vi "Frequency_Counter_BK_SoftFP.vi"(0 "reference in":refnum<class "Frequency_Counter_BK.lvclass">, 2 "Floating":bool, 5 "error in (no error)":errorcluster) -> (14 "reference out":refnum<class "Frequency_Counter_BK.lvclass">, 19 "error out":errorcluster)   [LabVIEW 2022 SP3, in "Frequency_Counter_BK.lvlib" / "Frequency_Counter_BK.lvclass"]
uses:
  Frequency_Counter_BK.lvclass
  Components/ViPER.lvlibp/ViPER.lvclass
  C:/Projects/Medulla/ViPER/Examples/Flux_Capacitor_Tester/Components/ViPER.lvlibp/ViPER.lvclass
panel:
  in  "Connect":bool
  out "Freq MHz":dbl format="%.4f"
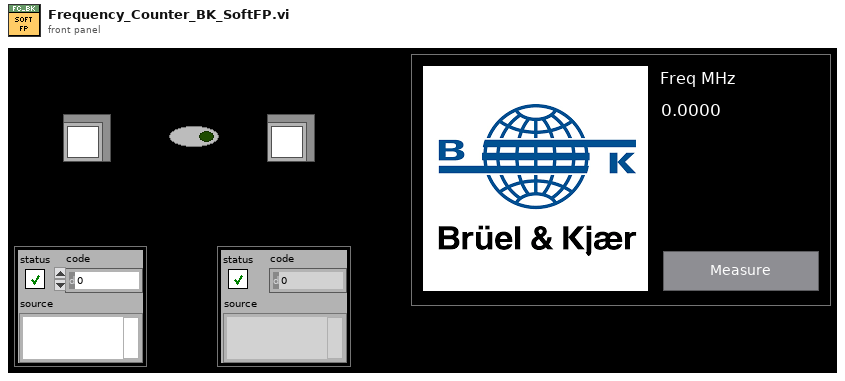
[diagram p1: front panel]
types:
  T1 = enum32{"Invalid", "Standard", "Closed", "Hidden", "Minimized", "Maximized"}
  T2 = typedef "Frequency_Counter_BK.lvlib/Frequency_Counter_BK.lvclass/ObjectAttributes.ctl" = cluster{"Config":T3, "Freq":dbl}
  T3 = typedef "Frequency_Counter_BK.lvlib/Frequency_Counter_BK.lvclass/Config.ctl" = cluster{"ComPort":refnum<visa-resource-name>, "Function":i8, "Gate_Time":i8}
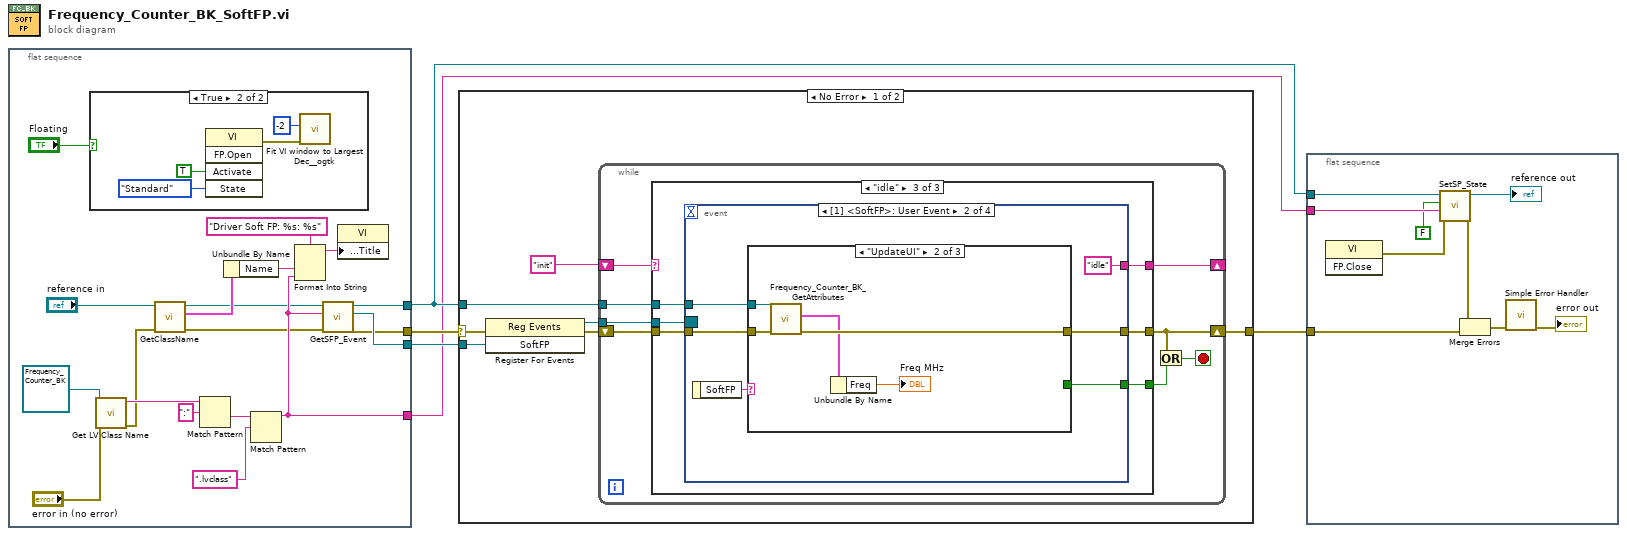
[diagram p0: block diagram]
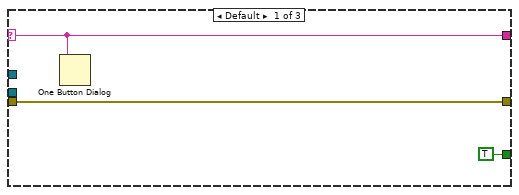
[diagram p3: hidden frame]
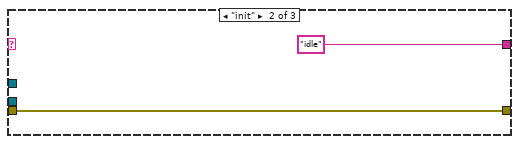
[diagram p4: hidden frame]
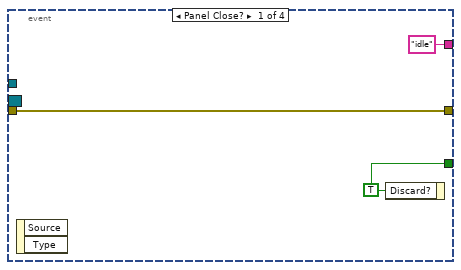
[diagram p5: hidden frame]
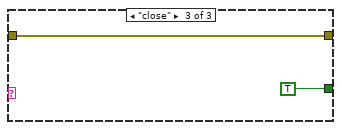
[diagram p7: hidden frame]
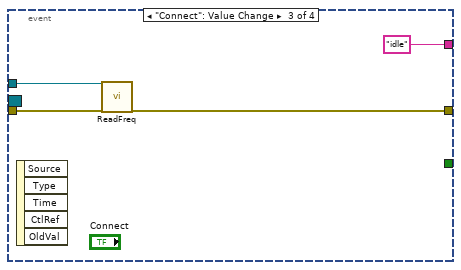
[diagram p8: hidden frame]
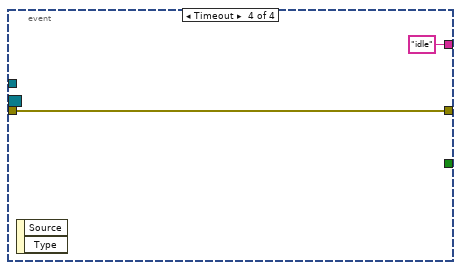
[diagram p9: hidden frame]
diagram:
  n1 = flat-sequence {
    tunnel: [w21] -> w5
    tunnel: [w20] -> w2
    tunnel: [w24] -> w3
    tunnel: [w12] -> w1
    frame #0 {
      n2 = case shown="True" "Floating" {
        frame False {
        }
        frame True {
          n3 = invoke class="VI" method="FP.Open"("Activate"=TRUE ("Activate?"), "State"=T1."Standard") -> (error out=w25:errorcluster)  [unwired: 3 in, 4 out]
          n4 = call <userlib>:"Fit VI window to Largest Dec__ogtk.vi"("error in (no error)"=w25, "border spacing (2 px)"=-2) -> ()  [unwired: 4 in, 2 out]
        }
      }
      n5 = call <vilib>:"Get LV Class Name.vi"("error in (no error)"="error in (no error)", "object"=refnum<class "Frequency_Counter_BK.lvclass"> refnum ("reference")) -> ("error out"=w11:errorcluster, "class name"=w17:string)  [unwired: 8 in]
      n6 = call "GetClassName.vi"("error in (no error)"=w11, "reference in"="reference in") -> ("error out"=w10:errorcluster, "Details"=w9:cluster{"Name":string, "Class":string}, "reference out"=w7:refnum<class "Frequency_Counter_BK.lvclass">)  [unwired: 7 in]
      n7 = Match Pattern(string=w17, regular expression=":") -> (after substring=w15:string)  [unwired: 1 in, 3 out]
      n8 = Unbundle By Name(w9) -> ("Name"=w19:string)
      n9 = Match Pattern(string=w15, regular expression=".lvclass") -> (before substring=w12:string)  [unwired: 1 in, 3 out]
      n10 = Format Into String(format string="Driver Soft FP: %s: %s", w19, w12) -> (resulting string=w23:string)  [unwired: 2 in, 1 out]
      n11 = call-dynamic "GetSFP_Event.vi"("error in (no error)"=w10, "Ancestor"=w12, "reference in"=w7) -> ("error out"=w21:errorcluster, "SoftFP"=w24:refnum<user-event>, "reference out"=w20:refnum<class "Frequency_Counter_BK.lvclass">)  [unwired: 6 in]
      n12 = property class="VI"("Front Panel.Title"=w23) -> ()  [unwired: 2 in, 2 out]
    }
  }
  n13 = case shown="No Error" w5 {
    selector: w5 -> [w33 w78]
    tunnel: [w29 w78] -> w4
    tunnel: w2 -> [w30 _]
    tunnel: w3 -> [w35 _]
    frame No Error {
      n14 = register-events(error in=w33, w35) -> (reference out=w34:refnum<event-registration>, error out=w32:errorcluster)  [unwired: 1 in]
      n15 = while {
        shift-right: [w40] -> w29
        shift-left: w32 -> [w43]
        tunnel: w34 -> [w42]
        tunnel: w30 -> [w41]
        shift-right: [w36] -> _
        shift-left: "init" -> [w37]
        stop <- w39 stop-if-true
        n16 = case shown="\"idle\"" w37 {
          selector: w37 -> [w44 _ _]
          tunnel: w43 -> [w45 w47 w54]
          tunnel: w42 -> [_ _ w53]
          tunnel: w41 -> [_ _ w52]
          tunnel: [w45 w47 w51] -> w40
          tunnel: [TRUE ("Discard?") _ w50] -> w38
          tunnel: [w44 "idle" w49] -> w36
          frame Default {
            n17 = One Button Dialog(message=w44) -> ()  [unwired: 1 in, 1 out]
          }
          frame "init" {
          }
          frame "idle" {
            n18 = event shown="[1] <SoftFP>: User Event" {
              selector: w53 -> [_ _ _ _]
              dyn-events: _ -> [_ _ _ _]
              timeout: _ -> [_ _ _ _]
              tunnel: w54 -> [w57 w63 w75 w77]
              tunnel: [w57 w61 w74 w77] -> w51
              tunnel: [w56 w60 _ _] -> w50
              tunnel: w52 -> [_ w58 w73 _]
              tunnel: ["idle" "idle" "idle" "idle"] -> w49
              event Panel Close? {
                w56 = TRUE ("Discard?")
                n19 = event-data() -> ()  [unwired: 1 in, 2 out]
                n20 = event-data("Discard?"=w56) -> ()  [unwired: 1 in, 1 out]
              }
              event User Event {
                n21 = event-data() -> ("SoftFP"=w62:string)  [unwired: 1 in]
                n22 = case shown="\"UpdateUI\"" w62 {
                  tunnel: w63 -> [w64 w69 w71]
                  tunnel: [w64 w67 w71] -> w61
                  tunnel: [_ _ TRUE ("Discard?")] -> w60
                  tunnel: w58 -> [_ w68 _]
                  frame Default {
                  }
                  frame "UpdateUI" {
                    n23 = call "Frequency_Counter_BK_GetAttributes.vi"("error in (no error)"=w69, "reference in"=w68) -> ("error out"=w67:errorcluster, "Data"=w66:T2)  [unwired: 6 in, 2 out]
                    n24 = Unbundle By Name(w66) -> ("Freq"=→"Freq MHz":dbl)
                  }
                  frame "close" {
                  }
                }
              }
              event "Connect": Value Change {
                n25 = event-data() -> ()  [unwired: 1 in, 5 out]
                n26 = call-dynamic "ReadFreq.vi"("reference in"=w73, "error in (no error)"=w75) -> ("error out"=w74:errorcluster)  [unwired: 15 in, 2 out]
              }
              event Timeout {
                n27 = event-data() -> ()  [unwired: 1 in, 2 out]
              }
            }
          }
        }
        n28 = Or(x=w40, y=w38) -> (x .or. y?=w39:bool)
      }
    }
    frame Error {
    }
  }
  n29 = flat-sequence {
    tunnel: w4 -> [w85]
    tunnel: w2 -> [w80]
    tunnel: w1 -> [w82]
    frame #0 {
      n30 = invoke class="VI" method="FP.Close"() -> (error out=w84:errorcluster)  [unwired: 3 in, 2 out]
      n31 = call "SetSP_State.vi"("error in (no error)"=w84, "Ancestor"=w82, "SP Open"=FALSE, "reference in"=w80) -> ("error out"=w83:errorcluster, "reference out"=→"reference out":refnum<class "Frequency_Counter_BK.lvclass">)  [unwired: 6 in]
      n32 = Merge Errors(w83, w85) -> (w87:errorcluster)
      n33 = call <vilib>:"Simple Error Handler.vi"("error in (no error)"=w87) -> ("error out"=→"error out":errorcluster)  [unwired: 4 in, 4 out]
    }
  }
